vi "VI_RemoveAllBreakpoints.vi"(7 "Target":T1=enum."Caller VI from Menu", 8 "Error In":errorcluster) -> (0 "Error Out":errorcluster)   [LabVIEW 2014]
uses:
  <vilib>/Utility/miscctls.llb/LVBreakpointStatusEnum.ctl
  <vilib>/Utility/miscctls.llb/LVPointTypeDef.ctl
  Project_VI_WhichTarget_Selector.ctl
panel:
  out "Progress Bar":u8(slide) scale=0.0..100.0
  out "Number of VIs to check":string
  out "wires and nodes checked":i64
  out "diagrams checked":i64
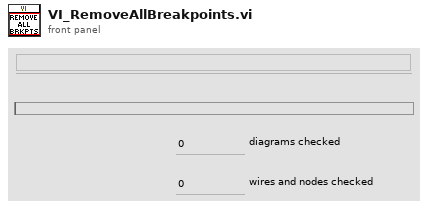
[diagram p1: front panel]
types:
  T1 = typedef "Project_VI_WhichTarget_Selector.ctl" = enum16{"All VIs in App", "Caller VI from Menu"}
  T2 = typedef "LVPointTypeDef.ctl" = cluster{"Horizontal":i16, "Vertical":i16}
  T3 = typedef "LVBreakpointStatusEnum.ctl" = enum8{"Cleared Break", "Enabled Break", "Disabled Break"}
  T4 = enum32{"Invalid", "Standard", "Closed", "Hidden", "Minimized", "Maximized"}
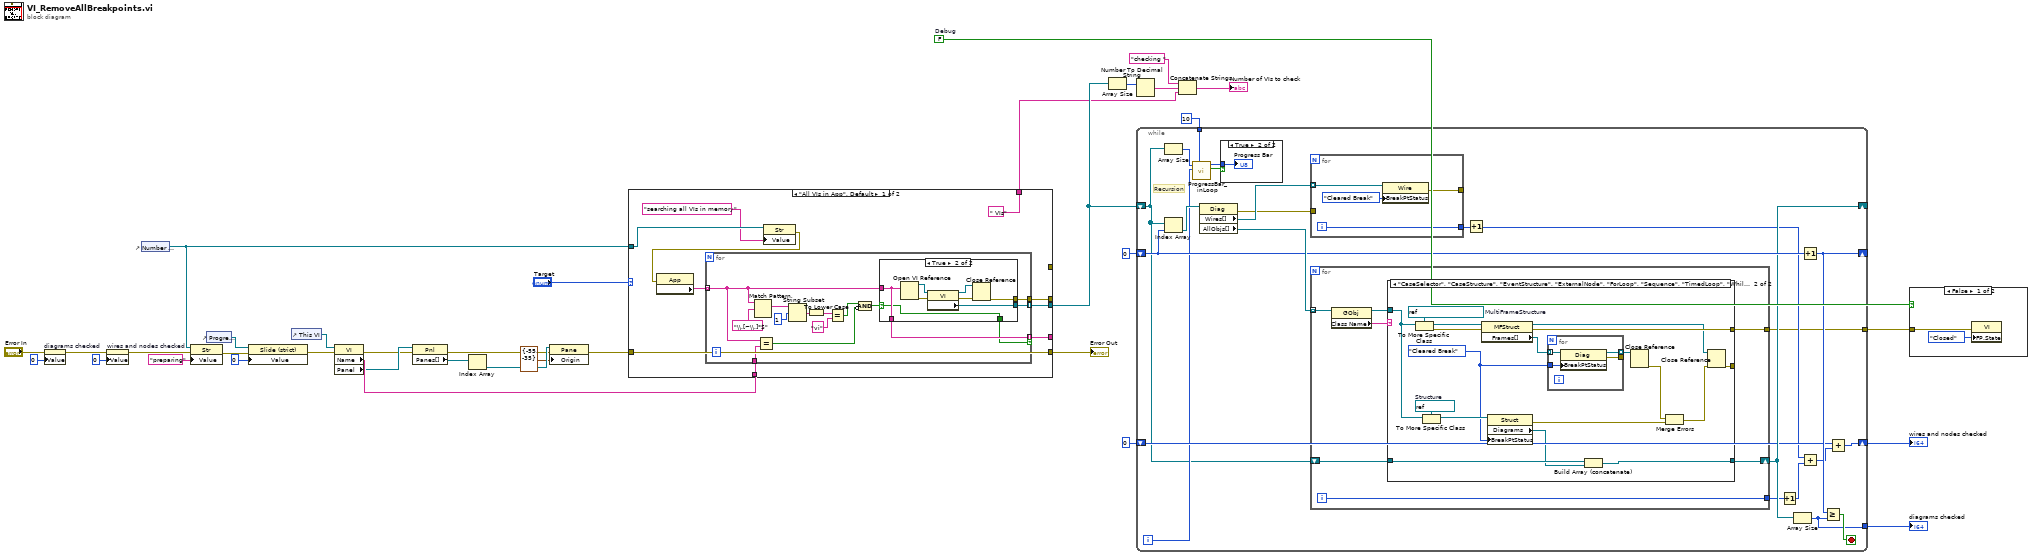
[diagram p0: block diagram]
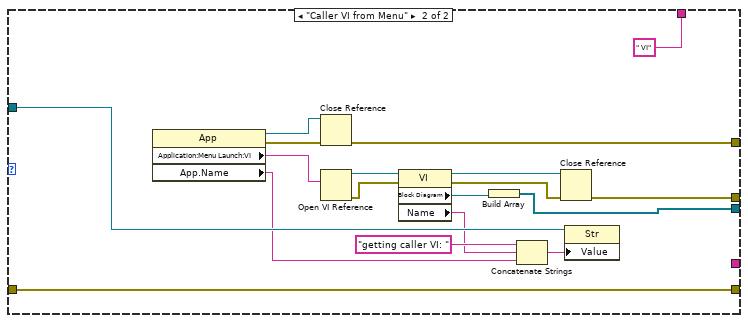
[diagram p4: hidden frame]
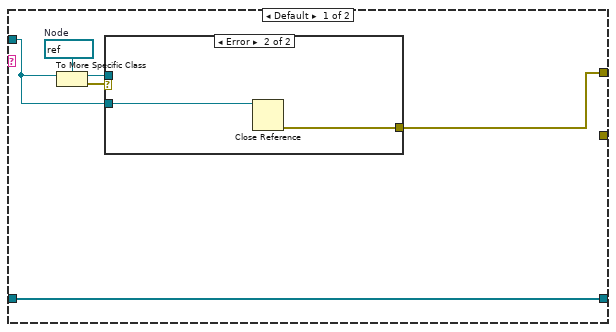
[diagram p6: hidden frame]
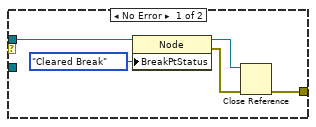
[diagram p7: hidden frame]
diagram:
  w10 = FALSE  # Debug
  n1 = property on="diagrams checked" class="DigNum (strict)"(error in="Error In", "Value"=i64 0 ("diagrams checked")) -> (error out=w6:errorcluster)  [unwired: 1 in, 1 out]
  n2 = property on="wires and nodes checked" class="DigNum (strict)"(error in=w6, "Value"=i64 0 ("diagrams checked")) -> (error out=w5:errorcluster)  [unwired: 1 in, 1 out]
  n3 = control-ref of="Number of VIs to check"() -> (w9:refnum<vi>)
  n4 = property class="Str"(reference=w9, error in=w5, "Value"="preparing") -> (error out=w4:errorcluster)  [unwired: 1 out]
  n5 = control-ref of="Progress Bar"() -> (w13:refnum<vi>)
  n6 = property class="Slide (strict)"(reference=w13, error in=w4, "Value"=u8 0) -> (error out=w14:errorcluster)  [unwired: 1 out]
  n7 = control-ref of="This VI"() -> (w22:refnum<vi>)
  n8 = property class="VI"(reference=w22, error in=w14) -> (error out=w15:errorcluster, "Name"=w33:string, "Panel"=w17:refnum<vi>)  [unwired: 1 out]
  n9 = property class="Pnl"(reference=w17, error in=w15) -> (error out=w16:errorcluster, "Panes[]"=w21:refnum<vi>[])  [unwired: 1 out]
  n10 = Index Array(array=w21) -> (element=w20:refnum<vi>)  [unwired: 1 in]
  n11 = property class="Pane"(reference=w20, error in=w16, "Origin"=T2 {"Horizontal"=-55, "Vertical"=-35}) -> (error out=w19:errorcluster)  [unwired: 1 out]
  n12 = case shown="\"All VIs in App\", Default" "Target" {
    tunnel: [w44 w79] -> w30
    tunnel: [w43 _] -> _
    tunnel: [w41 w78] -> _
    tunnel: w33 -> [w42 _]
    tunnel: [_ w77] -> _
    tunnel: [w40 w76] -> w26
    tunnel: w19 -> [w40 w76]
    tunnel: w9 -> [w39 w75]
    tunnel: [" VIs" ("string") " VI" ("string")] -> w25
    frame "All VIs in App", Default {
      n13 = property class="Str"(reference=w39, "Value"="searching all VIs in memory" ("string")) -> (error out=w37:errorcluster)  [unwired: 1 in, 1 out]
      n14 = property class="App"(error in=w37) -> ("Application:All VIs In Memory"=w45:string[])  [unwired: 1 in, 2 out]
      n15 = for {
        tunnel: w45 -> [w53] mode=indexing
        tunnel: [w60] -> w44 mode=indexing
        tunnel: [w55] -> w43 mode=indexing if=w54
        tunnel: w42 -> [w52]
        tunnel: [w46] -> w41
        n16 = Match Pattern(string=w53, regular expression="\\.[~\\.]*$") -> (match substring=w59:string)  [unwired: 4 out]
        n17 = Equal?(x=w53, y=w52) -> (x = y?=w51:bool)
        n18 = String Subset(string=w59, offset (0)=1) -> (substring=w56:string)  [unwired: 1 out]
        n19 = To Lower Case(string=w56) -> (all lower case string=w49:string)
        n20 = Equal?(x=w49, y="vi") -> (x = y?=w47:bool)
        n21 = Compound Arithmetic op=AND(w47, invert w51) -> (w50:bool)
        n22 = case shown="True" w50 {
          selector: w50 -> [w61 w62]
          tunnel: [_ w67] -> w60
          tunnel: w53 -> [_ w65]
          tunnel: [_ w65] -> w55
          tunnel: [w61 w62] -> w54
          tunnel: [_ w64] -> w46
          frame False {
          }
          frame True {
            n23 = Open VI Reference(vi path=w65) -> (vi reference=w69:refnum<vi>, error out=w68:errorcluster)  [unwired: 5 in]
            n24 = property class="VI"(reference=w69, error in=w68) -> (reference out=w66:refnum<vi>, error out=w63:errorcluster, "Block Diagram"=w67:refnum<vi>)
            n25 = Close Reference(reference=w66, error in (no error)=w63) -> (error out=w64:errorcluster)
          }
        }
      }
    }
    frame "Caller VI from Menu" {
      n26 = property class="App"() -> (reference out=w80:refnum<vi>, error out=w81:errorcluster, "Application:Menu Launch:VI"=w87:string, "App.Name"=w70:string)  [unwired: 2 in]
      n27 = Close Reference(reference=w80, error in (no error)=w81) -> (error out=w77:errorcluster)
      n28 = Open VI Reference(vi path=w87) -> (vi reference=w85:refnum<vi>, error out=w86:errorcluster)  [unwired: 5 in]
      n29 = property class="VI"(reference=w85, error in=w86) -> (reference out=w82:refnum<vi>, error out=w83:errorcluster, "Block Diagram"=w84:refnum<vi>, "Name"=w73:string)
      n30 = Build Array(w84) -> (w79:refnum<vi>[])
      n31 = Concatenate Strings("getting caller VI: " ("string"), w73, w70) -> (w72:string)
      n32 = Close Reference(reference=w82, error in (no error)=w83) -> (error out=w78:errorcluster)
      n33 = property class="Str"(reference=w75, "Value"=w72) -> ()  [unwired: 1 in, 2 out]
    }
  }
  "Error Out" <- w26
  n34 = Array Size(array=w30) -> (size(s)=w24:i32)
  n35 = Number To Decimal String(number=w24) -> (decimal integer string=w29:string)  [unwired: 1 in]
  n36 = while {
    shift-right: [w106] -> _
    shift-left: w30 -> [w89]
    shift-right: [w105] -> _
    shift-left: 0 ("index") -> [w107]
    shift-right: [w103] -> w32
    shift-left: 0 ("index") -> [w100]
    tunnel: [w96] -> w31
    tunnel: 10 ("every nth iteration") -> [w94]
    tunnel: [w90] -> w11
    i -> [w93]
    stop <- w104 stop-if-true
    # "Recursion"
    n37 = Array Size(array=w89) -> (size(s)=w88:i32)
    n38 = Index Array(array=w89, index=w107) -> (element=w108:refnum<vi>)
    n39 = call "ProgressBar_inLoop.vi"("every nth iteration"=w94, "current iteraion (In)"=w93, "Number of Loops (Total)"=w88) -> ("update control"=w91:bool, "Progress Bar"=w92:u8)  [unwired: 7 in]
    n40 = property class="Diag"(reference=w108) -> (error out=w95:errorcluster, "Wires[]"=w109:refnum<vi>[], "AllObjs[]"=w110:refnum<vi>[])  [unwired: 1 in, 1 out]
    n41 = case shown="True" w91 {
      tunnel: w92 -> [_ w111]
      frame False {
      }
      frame True {
        "Progress Bar" <- w111
      }
    }
    n42 = for {
      tunnel: w109 -> [w115] mode=indexing
      tunnel: [w113] -> w102
      tunnel: [w112] -> _
      tunnel: w95 -> [_]
      i -> [w113]
      n43 = property class="Wire"(reference=w115, "BreakPtStatus"=LVBreakpointStatusEnum."Cleared Break" ("Breakpoint Status")) -> (error out=w112:errorcluster)  [unwired: 1 in, 1 out]
    }
    n44 = for {
      tunnel: w110 -> [w122] mode=indexing
      shift-right: [w119] -> w106
      shift-left: w89 -> [w118]
      tunnel: [w117] -> w101
      tunnel: [w116] -> w90
      i -> [w117]
      n45 = property class="GObj"(reference=w122) -> (reference out=w120:refnum<vi>, "Class Name"=w121:string)  [unwired: 1 in, 1 out]
      n46 = case shown="\"CaseSelector\", \"CaseStructure\", \"EventStructure\", \"ExternalNode\", \"ForLoop\", \"Sequence\", \"TimedLoop\", \"WhileLoop\"" w121 {
        tunnel: w120 -> [w124 w147]
        tunnel: w118 -> [w128 w152]
        tunnel: [w128 w151] -> w119
        tunnel: [w123 w142] -> w116
        tunnel: [_ w137] -> _
        frame Default {
          w127 = refnum<vi> refnum  # Node
          n47 = To More Specific Class(target class=w127, reference=w124) -> (specific class reference=w126:refnum<vi>, error out=w125:errorcluster)  [unwired: 1 in]
          n48 = case shown="Error" w125 {
            tunnel: w126 -> [w131 _]
            tunnel: w124 -> [_ w135]
            tunnel: [w133 w134] -> w123
            frame No Error {
              n49 = property class="Node"(reference=w131, "BreakPtStatus"=LVBreakpointStatusEnum."Cleared Break" ("Breakpoint Status")) -> (reference out=w130:refnum<vi>, error out=w129:errorcluster)  [unwired: 1 in]
              n50 = Close Reference(reference=w130, error in (no error)=w129) -> (error out=w133:errorcluster)
            }
            frame Error {
              n51 = Close Reference(reference=w135) -> (error out=w134:errorcluster)  [unwired: 1 in]
            }
          }
        }
        frame "CaseSelector", "CaseStructure", "EventStructure", "ExternalNode", "ForLoop", "Sequence", "TimedLoop", "WhileLoop" {
          w148 = refnum<vi> refnum  # MultiFrameStructure
          w144 = LVBreakpointStatusEnum."Cleared Break" ("Breakpoint Status")
          w153 = refnum<vi> refnum  # Structure
          n52 = To More Specific Class(target class=w148, reference=w147) -> (specific class reference=w146:refnum<vi>, error out=w143:errorcluster)  [unwired: 1 in]
          n53 = To More Specific Class(target class=w153, reference=w147) -> (specific class reference=w150:refnum<vi>)  [unwired: 1 in, 1 out]
          n54 = property class="MFStruct"(reference=w146, error in=w143) -> (reference out=w140:refnum<vi>, error out=w142:errorcluster, "Frames[]"=w145:refnum<vi>[])
          n55 = property class="Struct"(reference=w150, "BreakPtStatus"=w144) -> (error out=w139:errorcluster, "Diagrams"=w149:refnum<vi>[])  [unwired: 1 in, 1 out]
          n56 = for {
            tunnel: w145 -> [w157] mode=indexing
            tunnel: [w156] -> _
            tunnel: w144 -> [w155]
            tunnel: [w154] -> w141 mode=indexing
            n57 = property class="Diag"(reference=w157, "BreakPtStatus"=w155) -> (reference out=w154:refnum<vi>, error out=w156:errorcluster)  [unwired: 1 in]
          }
          n58 = Build Array (concatenate)(w152, w149) -> (w151:refnum<vi>[])
          n59 = Close Reference(reference=w141) -> (error out=w136:errorcluster)  [unwired: 1 in]
          n60 = Merge Errors(w136, w139) -> (w138:errorcluster)
          n61 = Close Reference(reference=w140, error in (no error)=w138) -> (error out=w137:errorcluster)
        }
      }
    }
    n62 = Increment(x=w102) -> (x+1=w99:i32)
    n63 = Increment(x=w101) -> (x+1=w98:i32)
    n64 = Array Size(array=w106) -> (size(s)=w96:i32)
    n65 = Increment(x=w107) -> (x+1=w105:i32)
    n66 = Add(x=w99, y=w98) -> (x+y=w97:i32)
    n67 = Greater Or Equal?(x=w105, y=w96) -> (x >= y?=w104:bool)
    n68 = Add(x=w100, y=w97) -> (x+y=w103:i32)
  }
  "diagrams checked" <- w31
  "wires and nodes checked" <- w32
  n69 = Concatenate Strings("checking " ("string"), w29, w25) -> (→"Number of VIs to check":string)
  n70 = case shown="False" w10 {
    tunnel: w11 -> [w159 _]
    frame False {
      n71 = property class="VI"(error in=w159, "FP.State"=T4."Closed" ("Front Panel Window:State")) -> ()  [unwired: 1 in, 2 out]
    }
    frame True {
    }
  }
